vi "aoc-2025-d04-1.vi"() -> ()   [LabVIEW 2020]
panel:
  in  "part 1":bool
  out "sum":i32
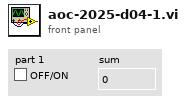
[diagram p1: front panel]
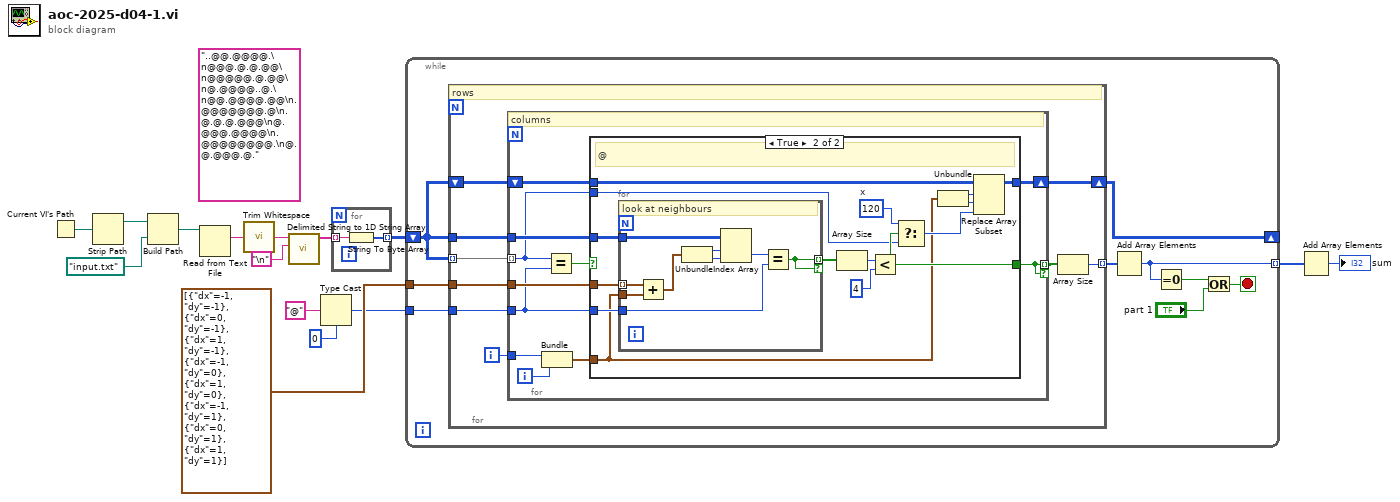
[diagram p0: block diagram]
diagram:
  (unwired) "..@@.@@@@.\n@@@.@.@.@@\n@@@@@.@.@@\n@.@@@@..@.\n@@.@@@@.@@\n.@@@@@@@.@\n.@.@.@.@@@\n@.@@@.@@@@\n.@@@@@@@@.\n@.@.@@@.@."
  n1 = Current VI's Path() -> (path=w6:path)
  n2 = Strip Path(path=w6) -> (stripped path=w5:path)  [unwired: 1 out]
  n3 = Build Path(base path=w5, name or relative path=path "input.txt") -> (appended path=w3:path)
  n4 = Read from Text File(file (use dialog)=w3) -> (text=w2:string)  [unwired: 3 in, 3 out]
  n5 = call <vilib>:"Trim Whitespace.vi"("string"=w2) -> ("trimmed string"=w14:string)  [unwired: 1 in]
  n6 = call <vilib>:"Delimited String to 1D String Array.vi"("delimiter"="\n", "delimited string"=w14) -> ("string array"=w13:string[])  [unwired: 9 in]
  n7 = Type Cast(type=u8 0, x="@") -> (*(type *) &x=w9:u8)
  n8 = for {
    tunnel: w13 -> [w17] mode=indexing
    tunnel: [w16] -> w7 mode=indexing
    n9 = String To Byte Array(string=w17) -> (unsigned byte array=w16:u8[])
  }
  n10 = while {
    tunnel: cluster{"dx":i32, "dy":i32}[] [{"dx"=-1, "dy"=-1}, {"dx"=0, "dy"=-1}, {"dx"=1, "dy"=-1}, {"dx"=-1, "dy"=0}, {"dx"=1, "dy"=0}, {"dx"=-1, "dy"=1}, {"dx"=0, "dy"=1}, {"dx"=1, "dy"=1}] -> [w26]
    tunnel: w9 -> [w25]
    tunnel: [w22] -> w8 mode=indexing
    shift-right: [w20] -> _
    shift-left: w7 -> [w23]
    stop <- w19 stop-if-true
    n11 = for {
      tunnel: w23 -> [w34]
      tunnel: w23 -> [w35] mode=indexing
      tunnel: w26 -> [w33]
      tunnel: w25 -> [w32]
      tunnel: [w27] -> w24 mode=indexing
      shift-right: [w29] -> w20
      shift-left: w23 -> [w30]
      i -> [w31]
      # "rows"
      n12 = for {
        tunnel: w35 -> [w36] mode=indexing
        tunnel: w34 -> [w46]
        tunnel: w33 -> [w45]
        tunnel: w32 -> [w40]
        tunnel: [w44] -> w28 mode=indexing if=w44
        tunnel: w31 -> [w42]
        shift-right: [w37] -> w29
        shift-left: w30 -> [w38]
        i -> [w43]
        # "columns"
        n13 = Bundle(w42, w43) -> (w41:cluster{i32, i32})  [unwired: 1 in]
        n14 = Equal?(x=w36, y=w40) -> (x = y?=w39:bool)
        n15 = case shown="True" w39 {
          tunnel: w46 -> [_ w62]
          tunnel: w45 -> [_ w61]
          tunnel: [_ w54] -> w44
          tunnel: w41 -> [_ w50]
          tunnel: w40 -> [_ w57]
          tunnel: w38 -> [w47 w55]
          tunnel: [w47 w56] -> w37
          tunnel: w36 -> [_ w52]
          frame False {
          }
          frame True {
            w53 = u8 120  # x
            # "@"
            n16 = for {
              tunnel: w62 -> [w71]
              tunnel: w61 -> [w65] mode=indexing
              tunnel: w57 -> [w67]
              tunnel: [w66] -> w60 mode=indexing if=w66
              tunnel: w50 -> [w64]
              # "look at neighbours"
              n17 = Add(x=w65, y=w64) -> (x+y=w63:cluster{i32, i32})
              n18 = Unbundle(w63) -> (w70:i32, w69:i32)
              n19 = Index Array(array=w71, index (row)=w70, index (col)=w69) -> (element=w68:u8)
              n20 = Equal?(x=w68, y=w67) -> (x = y?=w66:bool)
            }
            n21 = Array Size(array=w60) -> (size(s)=w59:i32)
            n22 = Less?(x=w59, y=4) -> (x < y?=w54:bool)
            n23 = Select(t=w53, s=w54, f=w52) -> (s? t:f=w51:u8)
            n24 = Unbundle(w50) -> (w49:i32, w48:i32)
            n25 = Replace Array Subset(array=w55, new element=w51, index (row)=w49, index (col)=w48) -> (w56:u8[][])
          }
        }
      }
      n26 = Array Size(array=w28) -> (size(s)=w27:i32)
    }
    n27 = Add Array Elements(numeric array=w24) -> (sum=w22:i32)
    n28 = Equal To 0?(x=w22) -> (x = 0?=w21:bool)
    n29 = Or(x=w21, y="part 1") -> (x .or. y?=w19:bool)
  }
  n30 = Add Array Elements(numeric array=w8) -> (sum=→"sum":i32)
